vi "GOOP_CopyLibraryClass.vi"(7 "ManualCopy":bool, 8 "error in":errorcluster, 9 "New Name":string, 10 "Path":path, 11 "LVClassIn":refnum<vi>) -> (0 "error out":errorcluster, 1 "New Lib Path":path, 3 "LVClassOut":refnum<vi>)   [LabVIEW 2012]
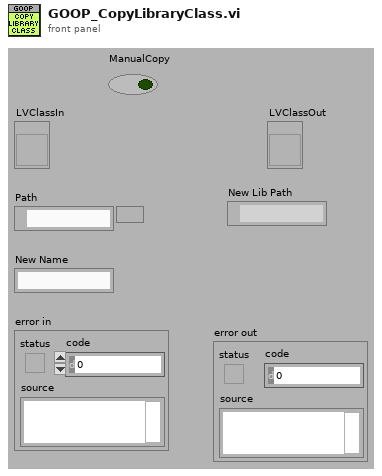
[diagram p1: front panel]
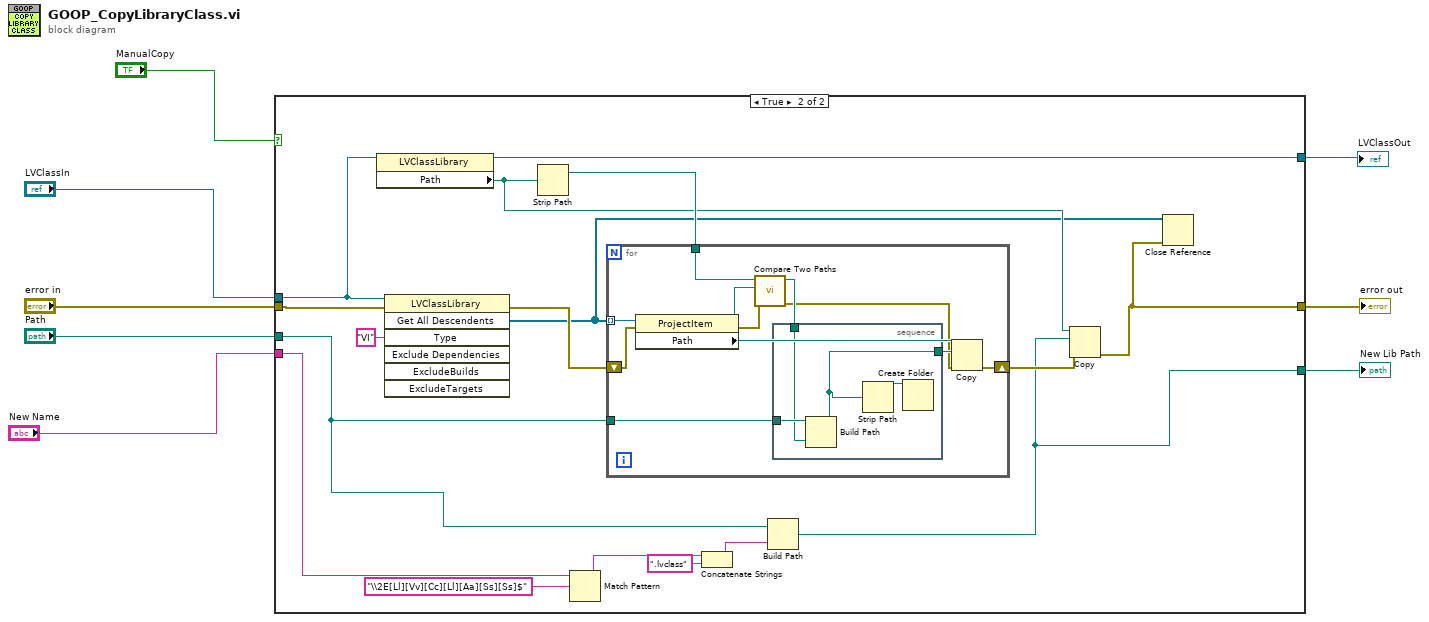
[diagram p0: block diagram]
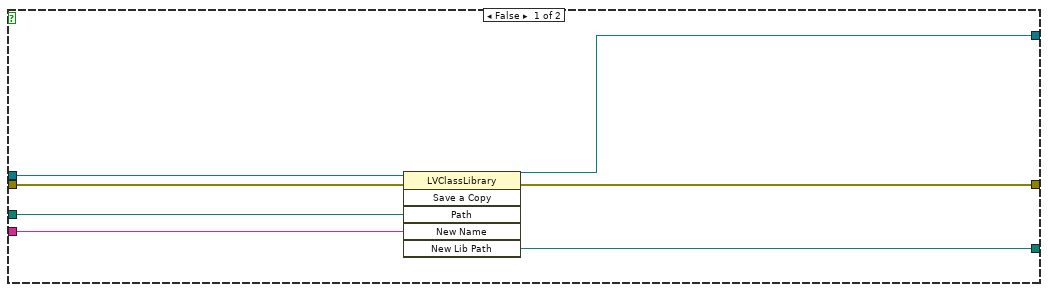
[diagram p2: hidden frame]
diagram:
  n1 = case shown="True" "ManualCopy" {
    tunnel: "error in" -> [w14 w27]
    tunnel: "LVClassIn" -> [w15 w26]
    tunnel: [w11 w17] -> w8
    tunnel: "New Name" -> [w12 w24]
    tunnel: "Path" -> [w13 w20]
    tunnel: [w10 w19] -> w6
    tunnel: [w9 w18] -> w1
    frame False {
      n2 = invoke class="LVClassLibrary" method="Save a Copy"(reference=w15, error in=w14, "Path"=w13, "New Name"=w12) -> (reference out=w9:refnum<vi>, error out=w11:errorcluster, "New Lib Path"=w10:path)  [unwired: 2 in, 3 out]
    }
    frame True {
      n3 = property class="LVClassLibrary"(reference=w26) -> (reference out=w18:refnum<vi>, "Path"=w30:path)  [unwired: 1 in, 1 out]
      n4 = invoke class="LVClassLibrary" method="Get All Descendents"(reference=w26, error in=w27, "Type"="VI") -> (error out=w28:errorcluster, "All Descendents"=w16:refnum<vi>[])  [unwired: 4 in, 5 out]
      n5 = Strip Path(path=w30) -> (stripped path=w31:path)  [unwired: 1 out]
      n6 = Match Pattern(string=w24, regular expression="\\2E[Ll][Vv][Cc][Ll][Aa][Ss][Ss]$") -> (before substring=w23:string)  [unwired: 1 in, 3 out]
      n7 = for {
        tunnel: w16 -> [w42] mode=indexing
        tunnel: w31 -> [w36]
        tunnel: w20 -> [w41]
        shift-right: [w39] -> w29
        shift-left: w28 -> [w37]
        n8 = property class="ProjectItem"(reference=w42, error in=w37) -> (error out=w38:errorcluster, "Path"=w35:path)  [unwired: 1 out]
        n9 = call <vilib>:"Compare Two Paths.vi"("error in (no error)"=w38, "Path 2"=w35, "Path 1"=w36) -> ("error out"=w33:errorcluster, "Relative Path from 1 to 2"=w40:path)  [unwired: 5 in, 2 out]
        n10 = stacked-sequence {
          tunnel: w41 -> [w46]
          tunnel: w40 -> [w45]
          tunnel: [w44] -> w34
          frame #0 {
            n11 = Build Path(base path=w46, name or relative path=w45) -> (appended path=w44:path)
            n12 = Strip Path(path=w44) -> (stripped path=w43:path)  [unwired: 1 out]
            n13 = Create Folder(path (use dialog)=w43) -> ()  [unwired: 2 in, 3 out]
          }
        }
        n14 = Copy(8:w33, 10:w34, 11:w35) -> (0:w39:errorcluster)  [unwired: 2 in, 2 out]
      }
      n15 = Concatenate Strings(w23, ".lvclass" ("string")) -> (w21:string)
      n16 = Build Path(base path=w20, name or relative path=w21) -> (appended path=w19:path)
      n17 = Copy(8:w29, 10:w19, 11:w30) -> (0:w17:errorcluster)  [unwired: 2 in, 2 out]
      n18 = Close Reference(reference=w16, error in (no error)=w17) -> ()  [unwired: 1 out]
    }
  }
  "error out" <- w8
  "New Lib Path" <- w6
  "LVClassOut" <- w1
